vi "kvCanObjBufAlloc.vi"(3 "error in (no error)":errorcluster, 4 "Object Type":bool, 5 "Channel Handle (input only)":i32) -> (0 "error out":errorcluster, 1 "Object Handle (output only)":i32, 2 "Channel Handle (output only)":i32)   [LabVIEW 2022 SP3]
doc: "Allocates an object buffer associated with the open handle to a CAN circuit.\n\nThe object can either be an Auto Response buffer or a Periodic buffer. Auto Response buffers transmit in response to an incoming message. Periodic buffers transmit at a configured frequency."
uses:
  canlib32.dll
panel:
  # "Auto Response"
  # "Periodic"
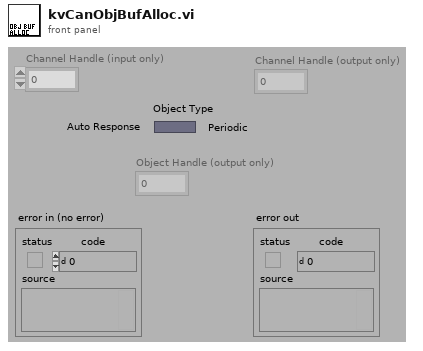
[diagram p1: front panel]
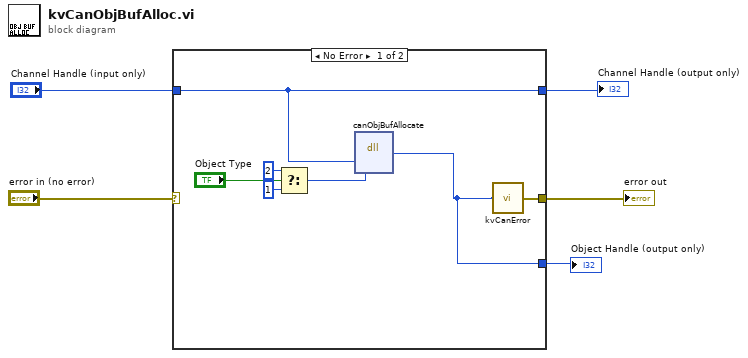
[diagram p0: block diagram]
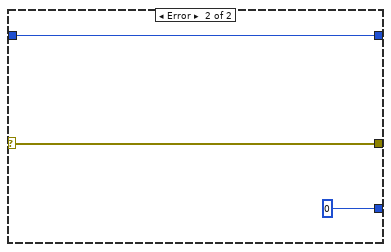
[diagram p2: hidden frame]
diagram:
  n1 = case shown="No Error" "error in (no error)" {
    selector: "error in (no error)" -> [_ w15]
    tunnel: [w7 w15] -> w4
    tunnel: "Channel Handle (input only)" -> [w9 w14]
    tunnel: [w9 w14] -> w2
    tunnel: [w6 0] -> w1
    frame No Error {
      n2 = Select(t=2, s="Object Type", f=1) -> (s? t:f=w8:i32)
      n3 = dll-call lib="canlib32.dll" fn="canObjBufAllocate"("chanNumber"=w9, "objType"=w8) -> (w6:i32)  [unwired: 5 in, 2 out]
      n4 = call "kvCanError.vi"("error code"=w6) -> ("error out"=w7:errorcluster)
    }
    frame Error {
    }
  }
  "Channel Handle (output only)" <- w2
  "error out" <- w4
  "Object Handle (output only)" <- w1
